vi "ExportPlots.vi"(11 "WaveformGraph in":refnum<vi>) -> ()   [LabVIEW 2022 SP3]
panel:
  in  "python":bool
  in  "matlab":bool
  in  "csv":bool
  # "Select file type to save"
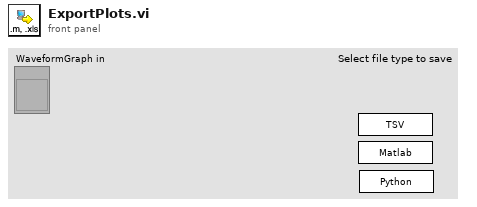
[diagram p1: front panel]
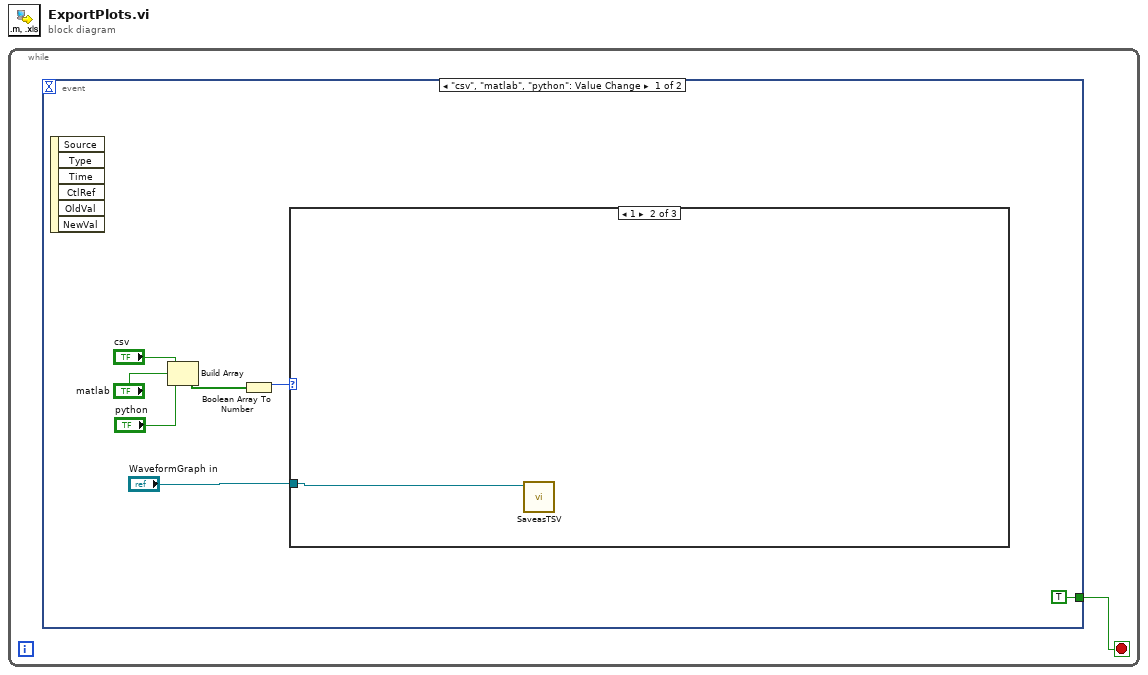
[diagram p0: block diagram]
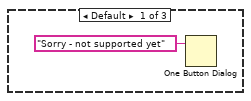
[diagram p2: hidden frame]
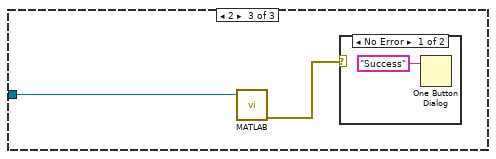
[diagram p3: hidden frame]
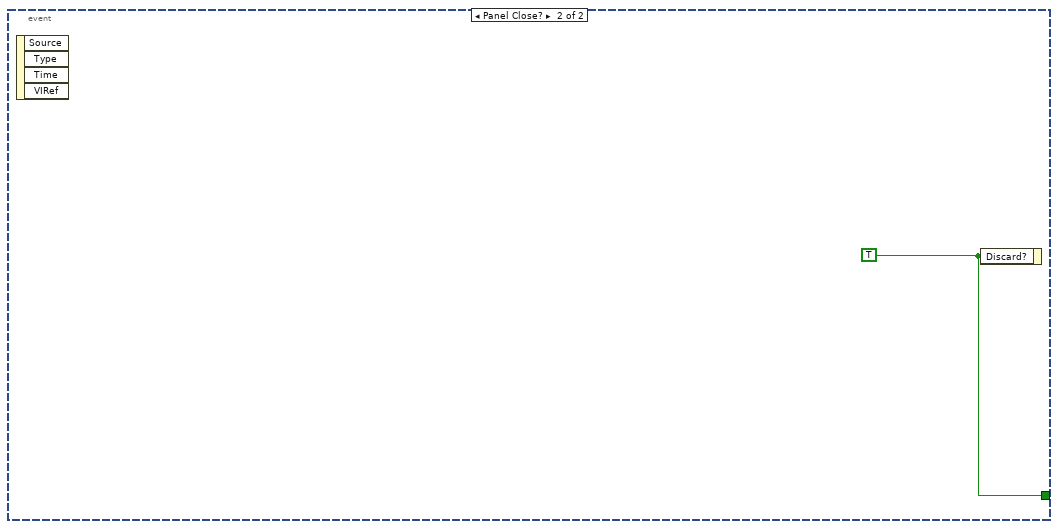
[diagram p5: hidden frame]
diagram:
  n1 = while {
    stop <- w1 stop-if-true
    n2 = event shown="[0] \"csv\", \"matlab\", \"python\": Value Change" {
      selector: _ -> [_ _]
      dyn-events: _ -> [_ _]
      timeout: _ -> [_ _]
      tunnel: [TRUE ("Discard?") w14] -> w1
      event "csv", "matlab", "python": Value Change {
        n3 = event-data() -> ()  [unwired: 1 in, 6 out]
        n4 = Build Array("csv", "matlab", "python") -> (w4:bool[])
        n5 = Boolean Array To Number(Boolean array=w4) -> (number=w3:u32)
        n6 = case shown="1" w3 {
          tunnel: "WaveformGraph in" -> [_ w10 w12]
          frame Default {
            n7 = One Button Dialog(message="Sorry - not supported yet") -> ()  [unwired: 1 in, 1 out]
          }
          frame 1 {
            n8 = call "SaveasTSV.vi"("Graph in"=w10) -> ()  [unwired: 11 in]
          }
          frame 2 {
            n9 = call "MATLAB.vi"("Graph"=w12) -> ("error out"=w11:errorcluster)  [unwired: 10 in]
            n10 = case shown="No Error" w11 {
              frame No Error {
                n11 = One Button Dialog(message="Success") -> ()  [unwired: 1 in, 1 out]
              }
              frame Error {
              }
            }
          }
        }
      }
      event Panel Close? {
        w14 = TRUE ("Discard?")
        n12 = event-data() -> ()  [unwired: 1 in, 4 out]
        n13 = event-data("Discard?"=w14) -> ()  [unwired: 1 in, 1 out]
      }
    }
  }
